vi "Drive_straight_command.vi"(9 "Fwd Bwd":dbl, 10 "Delay ms":u32=500, 11 "distance":dbl) -> ()   [LabVIEW 2014]
uses:
  TORC Code/GlobalVariable.vi
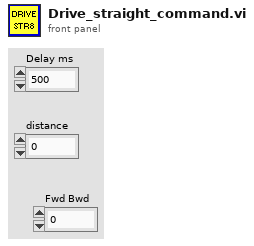
[diagram p1: front panel]
types:
  T1 = typedef "WPI_GyroDevRef.ctl" = cluster{"DevStatus":errorcluster, "Analog Module":T2, "Analog Channel":T3, "Offset":dbl, "Gain (VoltsPerDegree/Second)":dbl}
  T2 = typedef "FPGA_TypedefAnalogModule.ctl" = enum16{"Controller 1"}
  T3 = typedef "FPGA_AIChannel.ctl" = enum8{"AI 0", "AI 1", "AI 2", "AI 3", "AI MXP 0", "AI MXP 1", "AI MXP 2", "AI MXP 3", "Invalid"}
  T4 = typedef "WPI_EncoderDevRef.ctl" = cluster{"DevStatus":errorcluster, "EncoderIndex":T5, "CounterIndex":T6, "DistancePerCount":dbl, "Decoding Type":T7}
  T5 = typedef "FPGA_EncoderIdx.ctl" = enum8{"Enc 0", "Enc 1", "Enc 2", "Enc 3", "Enc 4", "Enc 5", "Enc 6", "Enc 7", "Invalid"}
  T6 = typedef "FPGA_CounterCtrSystemIndex.ctl" = enum8{"Ctr 0", "Ctr 1", "Ctr 2", "Ctr 3", "Ctr 4", "Ctr 5", "Ctr 6", "Ctr 7", "Invalid"}
  T7 = typedef "WPI_EncoderType.ctl" = enum16{"1x", "2x", "4x"}
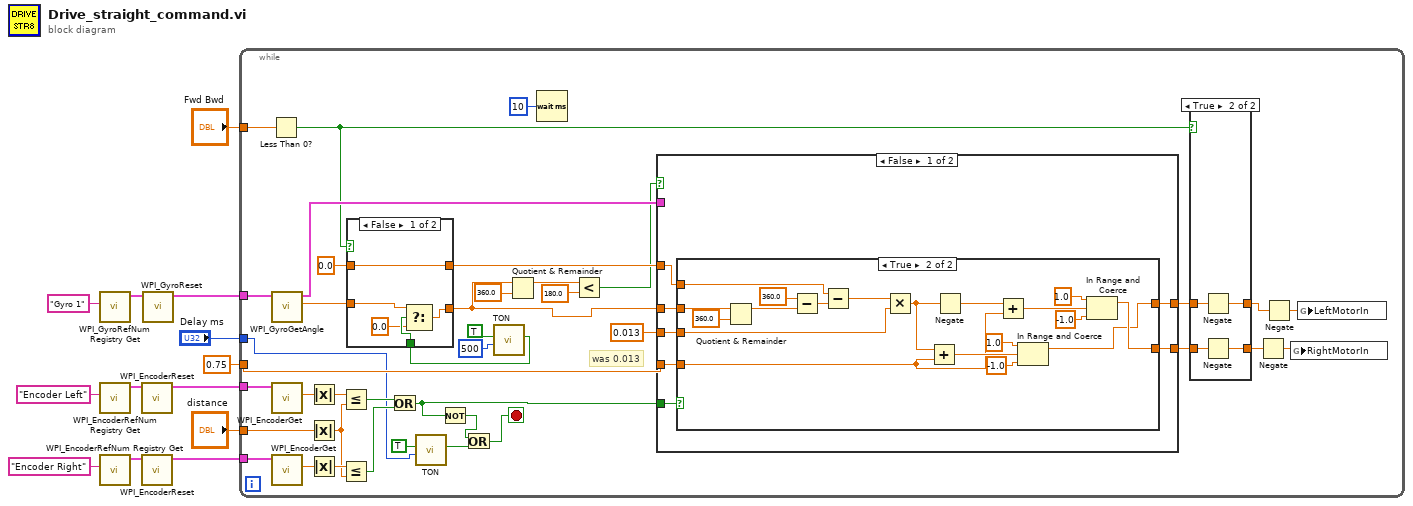
[diagram p0: block diagram]
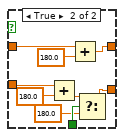
[diagram p3: hidden frame]
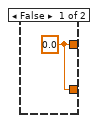
[diagram p4: hidden frame]
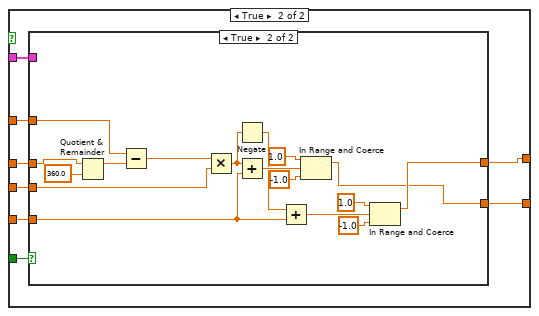
[diagram p5: hidden frame]
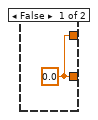
[diagram p6: hidden frame]
diagram:
  n1 = call <vilib>:"WPI_GyroRefNum Registry Get.vi"("refnum name"="Gyro 1") -> ("GyroDevRef"=w4:T1)  [unwired: 9 in, 1 out]
  n2 = call <vilib>:"WPI_EncoderRefNum Registry Get.vi"("refnum name"="Encoder Left") -> ("EncoderDevRef"=w12:T4)  [unwired: 9 in, 1 out]
  n3 = call <vilib>:"WPI_EncoderRefNum Registry Get.vi"("refnum name"="Encoder Right") -> ("EncoderDevRef"=w11:T4)  [unwired: 9 in, 1 out]
  n4 = call <vilib>:"WPI_EncoderReset.vi"("EncoderDevRef"=w12) -> ("EncoderDevRef"=w7:T4)  [unwired: 9 in, 1 out]
  n5 = call <vilib>:"WPI_EncoderReset.vi"("EncoderDevRef"=w11) -> ("EncoderDevRef"=w6:T4)  [unwired: 9 in, 1 out]
  n6 = call <vilib>:"WPI_GyroReset.vi"("GyroDevRef"=w4) -> ("GyroDevRef"=w3:T1)  [unwired: 9 in, 1 out]
  n7 = while {
    tunnel: 0.75 ("speed") -> [w43]
    tunnel: "distance" -> [w22]
    tunnel: w3 -> [w35]
    tunnel: w7 -> [w34]
    tunnel: w6 -> [w33]
    tunnel: "Fwd Bwd" -> [w32]
    tunnel: "Delay ms" -> [w28]
    stop <- w25 stop-if-true
    # "was 0.013"
    n8 = Less Than 0?(x=w32) -> (x < 0?=w15:bool)
    n9 = call <vilib>:"WPI_GyroGetAngle.vi"("GyroDevRef"=w35) -> ("Angle"=w45:dbl, "GyroDevRef"=w39:T1)  [unwired: 7 in, 2 out]
    n10 = call <vilib>:"WPI_EncoderGet.vi"("EncoderDevRef"=w34) -> ("Distance"=w44:dbl)  [unwired: 5 in, 5 out]
    n11 = call <vilib>:"WPI_EncoderGet.vi"("EncoderDevRef"=w33) -> ("Distance"=w50:dbl)  [unwired: 5 in, 5 out]
    n12 = Absolute Value(x=w44) -> (abs(x)=w51:dbl)
    n13 = Absolute Value(x=w22) -> (abs(x)=w52:dbl)
    n14 = Absolute Value(x=w50) -> (abs(x)=w53:dbl)
    n15 = Less Or Equal?(x=w51, y=w52) -> (x <= y?=w40:bool)
    n16 = Less Or Equal?(x=w53, y=w52) -> (x <= y?=w41:bool)
    n17 = Or(x=w40, y=w41) -> (x .or. y?=w19:bool)
    n18 = call "TON.vi"("Delay (ms)"=w28, "Input"=TRUE ("Digital_In")) -> ("Output"=w27:bool)  [unwired: 9 in]
    n19 = Not(x=w19) -> (.not. x?=w26:bool)
    n20 = Or(x=w26, y=w27) -> (x .or. y?=w25:bool)
    n21 = call "TON.vi"("Delay (ms)"=u32 500 ("Delay ms"), "Input"=TRUE ("Digital_In")) -> ("Output"=w20:bool)  [unwired: 9 in]
    n22 = case shown="False" w15 {
      tunnel: w45 -> [w63 w73]
      tunnel: [w62 w67] -> w21
      tunnel: 0.0 ("wanted angle") -> [w64 w69]
      tunnel: [w64 w71] -> w47
      tunnel: w20 -> [w61 w66]
      frame False {
        n23 = Select(t=w63, s=w61, f=0.0) -> (s? t:f=w62:dbl)
      }
      frame True {
        n24 = Add(x=w73, y=180.0) -> (x+y=w68:dbl)
        n25 = Add(x=w69, y=180.0) -> (x+y=w71:dbl)
        n26 = Select(t=w68, s=w66, f=180.0) -> (s? t:f=w67:dbl)
      }
    }
    n27 = Quotient & Remainder(x=w21, y=360.0) -> (x-y*floor(x/y)=w36:dbl)  [unwired: 1 out]
    n28 = Wait (ms)(milliseconds to wait=u32 10) -> ()  [unwired: 1 out]
    n29 = Less?(x=w36, y=180.0) -> (x < y?=w14:bool)
    n30 = case shown="False" w14 {
      tunnel: w47 -> [w79 w108]
      tunnel: [w75 w102] -> w49
      tunnel: w43 -> [w80 w107]
      tunnel: 0.013 ("Kp Gain") -> [w77 w106]
      tunnel: w19 -> [w76 w105]
      tunnel: [w74 w101] -> w48
      tunnel: w39 -> [_ w104]
      tunnel: w21 -> [w78 w103]
      frame False {
        n31 = case shown="True" w76 {
          tunnel: w80 -> [_ w88]
          tunnel: w79 -> [_ w93]
          tunnel: w78 -> [_ w92]
          tunnel: w77 -> [_ w87]
          tunnel: [w81 w84] -> w74
          tunnel: [w81 w83] -> w75
          frame False {
            w81 = 0.0
          }
          frame True {
            n32 = Quotient & Remainder(x=w92, y=360.0) -> (x-y*floor(x/y)=w90:dbl)  [unwired: 1 out]
            n33 = Subtract(x=360.0, y=w90) -> (x-y=w89:dbl)
            n34 = Subtract(x=w93, y=w89) -> (x-y=w82:dbl)
            n35 = Multiply(x=w82, y=w87) -> (x*y=w85:dbl)
            n36 = Add(x=w85, y=w88) -> (x+y=w97:dbl)
            n37 = Negate(x=w85) -> (-x=w86:dbl)
            n38 = Add(x=w86, y=w88) -> (x+y=w94:dbl)
            n39 = In Range and Coerce(upper limit=1.0, x=w97, lower limit=-1.0) -> (coerced(x)=w83:dbl)  [unwired: 1 out]
            n40 = In Range and Coerce(upper limit=1.0, x=w94, lower limit=-1.0) -> (coerced(x)=w84:dbl)  [unwired: 1 out]
          }
        }
      }
      frame True {
        n41 = case shown="True" w105 {
          tunnel: w104 -> [_ _]
          tunnel: w108 -> [_ w123]
          tunnel: [w109 w112] -> w102
          tunnel: w107 -> [_ w116]
          tunnel: w106 -> [_ w120]
          tunnel: [w109 w111] -> w101
          tunnel: w103 -> [_ w117]
          frame False {
            w109 = 0.0 ("output")
          }
          frame True {
            n42 = Quotient & Remainder(x=w117, y=360.0) -> (x-y*floor(x/y)=w124:dbl)  [unwired: 1 out]
            n43 = Subtract(x=w123, y=w124) -> (x-y=w110:dbl)
            n44 = Multiply(x=w110, y=w120) -> (x*y=w115:dbl)
            n45 = Negate(x=w115) -> (-x=w113:dbl)
            n46 = Add(x=w115, y=w116) -> (x+y=w121:dbl)
            n47 = Add(x=w113, y=w116) -> (x+y=w114:dbl)
            n48 = In Range and Coerce(upper limit=1.0, x=w121, lower limit=-1.0) -> (coerced(x)=w111:dbl)  [unwired: 1 out]
            n49 = In Range and Coerce(upper limit=1.0, x=w114, lower limit=-1.0) -> (coerced(x)=w112:dbl)  [unwired: 1 out]
          }
        }
      }
    }
    n50 = case shown="True" w15 {
      tunnel: w48 -> [w55 w59]
      tunnel: w49 -> [w54 w58]
      tunnel: [w55 w56] -> w30
      tunnel: [w54 w57] -> w31
      frame False {
      }
      frame True {
        n51 = Negate(x=w58) -> (-x=w56:dbl)
        n52 = Negate(x=w59) -> (-x=w57:dbl)
      }
    }
    n53 = Negate(x=w31) -> (-x=w16:dbl)
    n54 = Negate(x=w30) -> (-x=w17:dbl)
    n55 = global write "GlobalVariable.vi" "RightMotorIn"(w16) -> ()
    n56 = global write "GlobalVariable.vi" "LeftMotorIn"(w17) -> ()
  }
